vi "StringifiedData.vi"(8 "error in (no error)":errorcluster, 11 "PathMsg in":refnum<class "PathMsg.lvclass">) -> (0 "error out":errorcluster, 2 "Stringified Data":string, 3 "PathMsg out":refnum<class "PathMsg.lvclass">)   [LabVIEW 2013, in "LapDog.Messaging.v3.NativeTypes.lvlib" / "PathMsg.lvclass"]
doc: "This VI is used for the message probe. Child classes may override it and provide the message data in string format or a short string describing the data the message contains. This string will be displayed in the probe window."
uses:
  PathMsg.lvclass
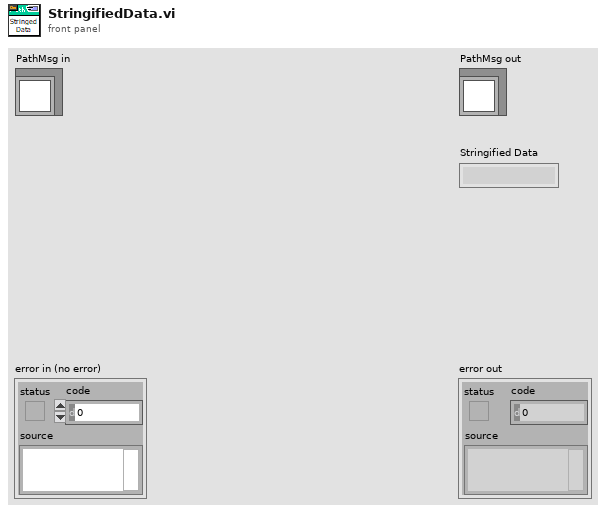
[diagram p1: front panel]
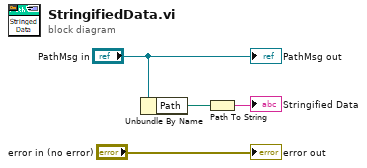
[diagram p0: block diagram]
diagram:
  n1 = Unbundle By Name("PathMsg in") -> ("Path"=w2:path)
  n2 = Path To String(path=w2) -> (string=→"Stringified Data":string)
  "error out" <- "error in (no error)"
  "PathMsg out" <- "PathMsg in"
